vi "Auto Hot Goal.vi"(10 "y":dbl[](array[numeric])=[156.0, 246.0, 258.0], 11 "x":dbl[](array[numeric])=[152.0, 48.0, 552.0]) -> (2 "x > y?":bool, 3 "element":dbl)   [LabVIEW 2013]
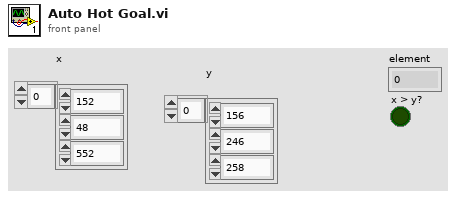
[diagram p1: front panel]
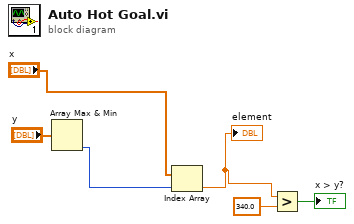
[diagram p0: block diagram]
diagram:
  n1 = Array Max & Min(array="y") -> (min index (indices)=w5:i32)  [unwired: 3 out]
  n2 = Index Array(array="x", index=w5) -> (element=w3:dbl)
  "element" <- w3
  n3 = Greater?(x=w3, y=340.0) -> (0:→"x > y?":bool)
